vi "Interference 1065.375 Textfile.vi"() -> (3 "Textfile":string[](array[string]))   [LabVIEW 2020, in "EPA 1065.lvlib" / "Interference verificaton 1065-375.lvlib"]
uses:
  Interference verificaton 1065-375.lvlib
  Sprachverwaltung/FGV Aktion Tabelle zerlegen.ctl
  Aktion FGV Interference.ctl
  Seiten/FT-IR/FGV FT-IR Aktionen.ctl
  Aktion Index uebersetzten.ctl
  Seiten/System Einstellungen V2/Aktioen FGV System Konstanten.ctl
  Visualisierungs Elemente/String - Ausgabefeld.ctl
  Seiten/FT-IR/FT-IR.lvlib
  Seiten/System Einstellungen V2/System Einstellungen V2.lvlib
  Sprachverwaltung/Sprachverwaltung.lvlib
panel:
  out "Tabellen-String":string
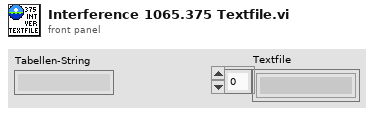
[diagram p1: front panel]
types:
  T1 = typedef "String - Ausgabefeld.ctl" = string
  T2 = typedef "System Einstellungen V2.lvlib/Aktioen FGV System Konstanten.ctl" = enum16{"lesen", "laden", "speichern", "Sprache"}
  T3 = typedef "EPA 1065.lvlib/Interference verificaton 1065-375.lvlib/Aktion Index uebersetzten.ctl" = enum16{"lesen", "schreiben", "auswerten"}
  T4 = typedef "FT-IR.lvlib/FGV FT-IR Aktionen.ctl" = enum16{"lesen", "NOG setzen", "NOS setzen", "Initialisieren", "speichern", "ALLES setzen", "FT-IR Spektrum loggen", "Komm Stoppen", "Spektrum LogKonfig"}
  T5 = typedef "EPA 1065.lvlib/Interference verificaton 1065-375.lvlib/Aktion FGV Interference.ctl" = enum16{"Lesen", "TestKonfig", "TestSetting", "Einheiten", "Ergebnis", "Laden", "Tabelle", "Speichern", "löschen"}
  T6 = typedef "Sprachverwaltung.lvlib/FGV Aktion Tabelle zerlegen.ctl" = enum16{"laden", "vereinzeln", "speichern"}
  T7 = typedef "EPA 1065.lvlib/Interference verificaton 1065-375.lvlib/TestSetting.ctl" = cluster{"Bearbeiter:":string, "Pfad:":path, "Textname:":string, "Analysator":T8}
  T8 = typedef "System Einstellungen V2.lvlib/Analysatoren.ctl" = string
  T9 = typedef "EPA 1065.lvlib/Interference verificaton 1065-375.lvlib/TestKonfig.ctl" = cluster{"Komponente:":u16, "Modus":T10, "CG Aufschaltzeit:":dbl, "Interferent 1:":u16, "Interferent 2:":u16, "Interferent 3:":u16, "Gasflaschen Nr.:":string, "Gasflaschen Nr.: 2":string, "Gasflaschen Nr.: 3":string, "Inter 1 aktiv":bool, "Inter 2 aktiv":bool, "Inter 3 aktiv":bool, "Accuracy":string, "Accuracy 2":string, "Accuracy 3":string, "Konzentration 1:":dbl, "Konzentration 2:":dbl, "Konzentration 3:":dbl}
  T10 = typedef "EPA 1065.lvlib/Interference verificaton 1065-375.lvlib/Modus.ctl" = u16
  T11 = typedef "EPA 1065.lvlib/Interference verificaton 1065-375.lvlib/Komponenten.ctl" = cluster{"Komponente":T1, "Komponente Index":i32, "Komponente 2":T1, "Komponente Index 2":i32, "Komponente 3":T1, "Komponente Index 3":i32, "Interferent 1":T1, "Interferent Index":i32, "Interferent 2":T1, "Interferent 2 Index":i32, "Interferent 3":T1, "Interferent 3 Index":i32, "Interferent 4":T1, "Interferent 4 Index":i32}
  T12 = cluster{"Modell":string, "ProjektNummer":string, "Software Version":string, "Seriennummer":string}
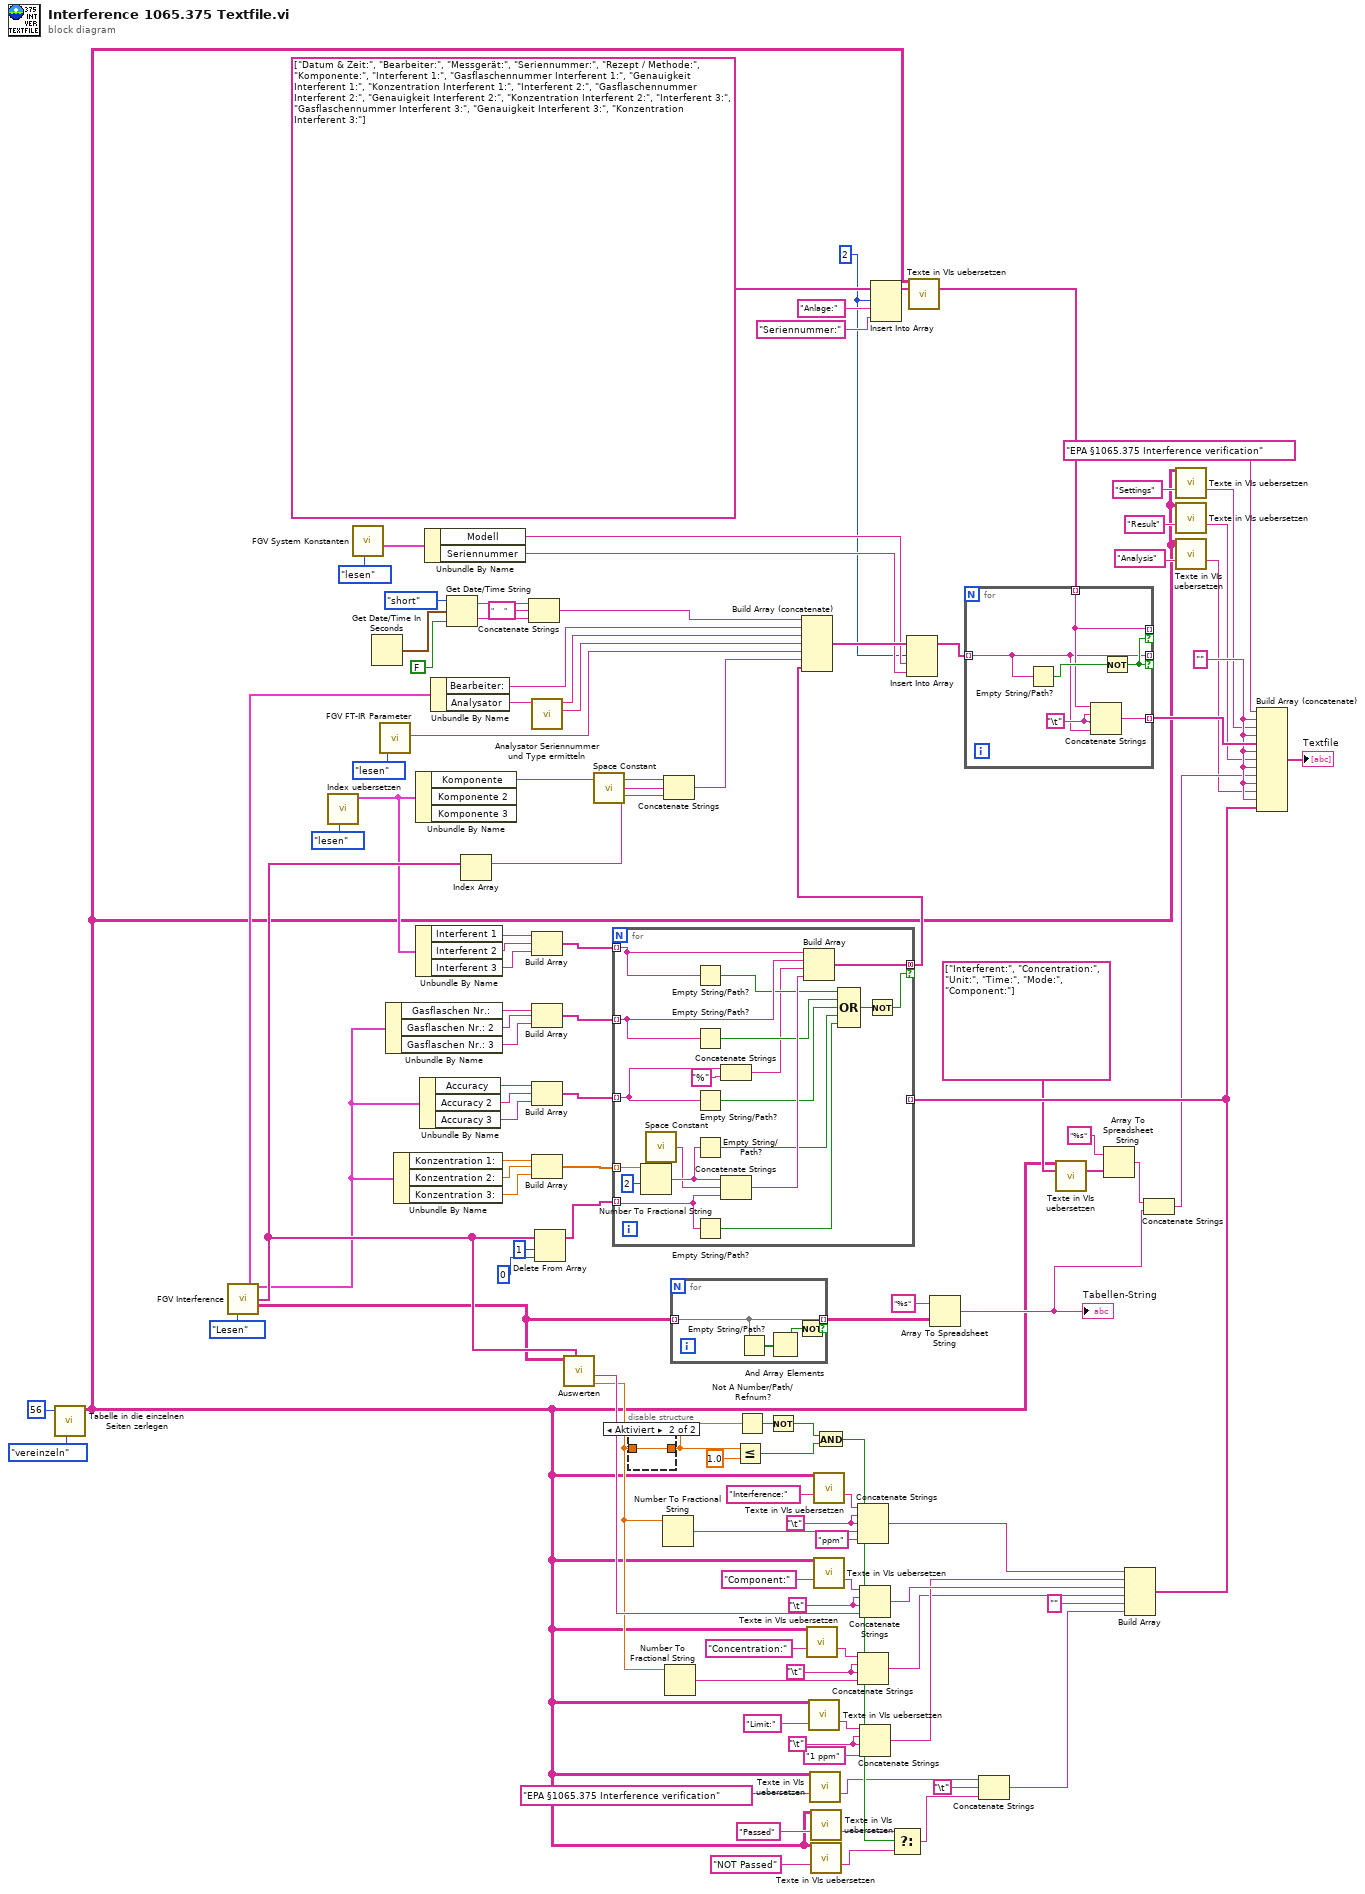
[diagram p0: block diagram]
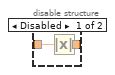
[diagram p2: hidden frame]
diagram:
  w35 = ""
  w52 = "\t"
  w53 = "\t"
  w54 = "\t"
  w55 = "\t"
  w63 = 2 ("Index")
  n1 = call "Tabelle in die einzelnen Seiten zerlegen.vi"("Aktion"=FGV_Aktion_Tabelle_zerlegen."vereinzeln", "Index (Seite)"=56) -> ("Sprachliste"=w4:string[][])  [unwired: 7 in, 2 out]
  n2 = call "FGV Interference.vi"("Aktion FGV Interference"=Aktion_FGV_Interference."Lesen") -> ("TestSetting"=w113:T7, "TestKonfig 2"=w82:T9, "Êinheiten"=w100:string[], "Tabelle"=w32:T1[][])  [unwired: 9 in, 2 out]
  n3 = call "Index uebersetzen.vi"("Aktion"=Aktion_Index_uebersetzten."lesen") -> ("Komponenten"=w95:T11)  [unwired: 9 in, 1 out]
  n4 = call "FGV System Konstanten.vi"("Aktionen"=Aktioen_FGV_System_Konstanten."lesen") -> ("Cluster out"=w72:T12)  [unwired: 6 in, 4 out]
  n5 = Get Date/Time In Seconds() -> (seconds since 1Jan1904=w112:timestamp)
  n6 = call "FGV FT-IR Parameter.vi"("Aktion"=FGV_FT-IR_Aktionen."lesen") -> ("Current Recipe"=w101:string)  [unwired: 11 in, 7 out]
  n7 = Unbundle By Name(w82) -> ("Gasflaschen Nr.:"=w94:string, "Gasflaschen Nr.: 2"=w93:string, "Gasflaschen Nr.: 3"=w92:string)
  n8 = Unbundle By Name(w82) -> ("Konzentration 1:"=w91:dbl, "Konzentration 2:"=w90:dbl, "Konzentration 3:"=w89:dbl)
  n9 = Unbundle By Name(w95) -> ("Komponente"=w75:T1)  [unwired: 2 out]
  n10 = Unbundle By Name(w95) -> ("Interferent 1"=w98:T1, "Interferent 2"=w97:T1, "Interferent 3"=w96:T1)
  n11 = Unbundle By Name(w82) -> ("Accuracy"=w81:string, "Accuracy 2"=w80:string, "Accuracy 3"=w79:string)
  n12 = Unbundle By Name(w72) -> ("Modell"=w65:string, "Seriennummer"=w64:string)
  n13 = Unbundle By Name(w113) -> ("Bearbeiter:"=w103:string, "Analysator"=w3:T8)
  n14 = Get Date/Time String(date format (0)=enum16{"short", "long", "abbreviated"}."short" ("Datumsformat (0)"), seconds (now)=w112, want seconds? (F)=FALSE ("Angabe von Sekunden? (F)")) -> (date string=w111:string, time string=w110:string)
  n15 = Index Array(array=w100) -> (element=w74:string)  [unwired: 1 in]
  n16 = Concatenate Strings(w111, "     " ("String"), w110) -> (w104:string)
  n17 = call "Analysator Seriennummer und Type ermitteln.vi"("Analysator"=w3) -> ("Type"=w2:string, "Name für Protokoll"=w1:string)  [unwired: 8 in, 1 out]
  n18 = Build Array(w98, w97, w96) -> (w88:T1[])
  n19 = Build Array(w94, w93, w92) -> (w87:string[])
  n20 = Build Array(w81, w80, w79) -> (w78:string[])
  n21 = Build Array(w91, w90, w89) -> (w86:dbl[])
  n22 = Delete From Array(array=w100, length=1 ("Länge"), index=0 ("Index")) -> (array with subset deleted=w84:string[])  [unwired: 1 out]
  n23 = call "Auswerten.vi"("Êinheiten"=w100, "Tabelle"=w32) -> ("Konzentration Komponente"=w49:dbl, "Komponente:"=w50:T1)  [unwired: 6 in, 2 out]
  n24 = call <vilib>:"Space Constant.vi"() -> ("String"=w76:string)
  n25 = disable-structure shown="Aktiviert" {
    disable-tunnel: w49 -> [w118 w119]
    disable-tunnel: [w117 w119] -> w45
    frame Disabled {
      n26 = Absolute Value(x=w118) -> (abs(x)=w117:dbl)
    }
    frame Enabled {
    }
  }
  n27 = Number To Fractional String(number=w49) -> (F-format string=w60:string)  [unwired: 3 in]
  n28 = Concatenate Strings(w75, w76, w74) -> (w102:string)
  n29 = Number To Fractional String(number=w49) -> (F-format string=w56:string)  [unwired: 3 in]
  n30 = for {
    tunnel: w32 -> [w123] mode=indexing
    tunnel: [w123] -> w33 mode=indexing if=w120
    n31 = Empty String/Path?(string/path=w123) -> (empty?=w122:bool[])
    n32 = And Array Elements(Boolean array=w122) -> (logical AND=w121:bool)
    n33 = Not(x=w121) -> (.not. x?=w120:bool)
  }
  n34 = Less Or Equal?(x=w45, y=1.0) -> (x <= y?=w43:bool)
  n35 = Not A Number/Path/Refnum?(number/path/refnum=w45) -> (NaN/Path/Refnum?=w44:bool)
  n36 = Not(x=w44) -> (.not. x?=w42:bool)
  n37 = call "Texte in VIs uebersetzen.vi"("Sprachliste"=w4, "String zum Übersetzen"="Concentration:" ("String")) -> ("String zum Übersetzen"=w13:string)  [unwired: 9 in, 4 out]
  n38 = call "Texte in VIs uebersetzen.vi"("Sprachliste"=w4, "String zum Übersetzen"="Limit:" ("String")) -> ("String zum Übersetzen"=w11:string)  [unwired: 9 in, 4 out]
  n39 = call "Texte in VIs uebersetzen.vi"("Sprachliste"=w4, "String zum Übersetzen"="EPA §1065.375 Interference verification") -> ("String zum Übersetzen"=w9:string)  [unwired: 9 in, 4 out]
  n40 = call "Texte in VIs uebersetzen.vi"("Sprachliste"=w4, "String zum Übersetzen"=T1 "Passed" ("String")) -> ("String zum Übersetzen"=w7:string)  [unwired: 9 in, 4 out]
  n41 = call "Texte in VIs uebersetzen.vi"("Sprachliste"=w4, "String zum Übersetzen"=T1 "NOT Passed" ("String")) -> ("String zum Übersetzen"=w5:string)  [unwired: 9 in, 4 out]
  n42 = call "Texte in VIs uebersetzen.vi"("Sprachliste"=w4, "String zum Übersetzen"="Interference:" ("String")) -> ("String zum Übersetzen"=w17:string)  [unwired: 9 in, 4 out]
  n43 = call "Texte in VIs uebersetzen.vi"("Sprachliste"=w4, "String zum Übersetzen"="Component:" ("String")) -> ("String zum Übersetzen"=w15:string)  [unwired: 9 in, 4 out]
  n44 = And(x=w42, y=w43) -> (x .and. y?=w61:bool)
  n45 = Concatenate Strings(w17, w55, w55, w60, "ppm" ("String")) -> (w58:string)
  n46 = Concatenate Strings(w13, w53, w53, w56) -> (w39:string)
  n47 = Concatenate Strings(w15, w54, w54, w50) -> (w57:string)
  n48 = Concatenate Strings(w11, w52, w52, "1 ppm" ("String")) -> (w40:string)
  n49 = Insert Into Array(array=string[] ["Datum & Zeit:", "Bearbeiter:", "Messgerät:", "Seriennummer:", "Rezept / Methode:", "Komponente:", "Interferent 1:", "Gasflaschennummer Interferent 1:", "Genauigkeit Interferent 1:", "Konzentration Interferent 1:", "Interferent 2:", "Gasflaschennummer Interferent 2:", "Genauigkeit Interferent 2:", "Konzentration Interferent 2:", "Interferent 3:", "Gasflaschennummer Interferent 3:", "Genauigkeit Interferent 3:", "Konzentration Interferent 3:"], index=w63, new element #1="Anlage:" ("Neues Element/Teil-Array"), new element #2="Seriennummer:" ("Neues Element/Teil-Array")) -> (w68:string[])
  n50 = Select(t=w7, s=w61, f=w5) -> (s? t:f=w19:string)
  n51 = call "Texte in VIs uebersetzen.vi"("Sprachliste"=w4, "String-Array zum Übersetzen"=w68) -> ("String-Array zum Übersetzen"=w77:string[])  [unwired: 9 in, 4 out]
  n52 = Array To Spreadsheet String(array=w33, 3:"%s" ("Format-String")) -> (spreadsheet string=w29:string)  [unwired: 1 in]
  "Tabellen-String" <- w29
  n53 = Concatenate Strings(w9, "\t", w19) -> (w37:string)
  n54 = call "Texte in VIs uebersetzen.vi"("Sprachliste"=w4, "String-Array zum Übersetzen"=string[] ["Interferent:", "Concentration:", "Unit:", "Time:", "Mode:", "Component:"]) -> ("String-Array zum Übersetzen"=w20:string[])  [unwired: 9 in, 4 out]
  n55 = Array To Spreadsheet String(array=w20, 3:"%s" ("Format-String")) -> (spreadsheet string=w30:string)  [unwired: 1 in]
  n56 = Build Array(w58, w40, w57, w39, "" ("Element"), w37) -> (w48:string[])
  n57 = for {
    tunnel: w88 -> [w139] mode=indexing
    tunnel: w87 -> [w138] mode=indexing
    tunnel: w86 -> [w142] mode=indexing
    tunnel: w84 -> [w141] mode=indexing
    tunnel: [w136] -> w83 mode=concatenating if=w124
    tunnel: w78 -> [w125] mode=indexing
    tunnel: w48 -> [_] mode=indexing
    n58 = Number To Fractional String(number=w142, precision (6)=i16 2 ("Genauigkeit (6)")) -> (F-format string=w140:string)  [unwired: 2 in]
    n59 = call <vilib>:"Space Constant.vi"() -> ("String"=w130:string)
    n60 = Empty String/Path?(string/path=w139) -> (empty?=w135:bool)
    n61 = Empty String/Path?(string/path=w138) -> (empty?=w134:bool)
    n62 = Empty String/Path?(string/path=w125) -> (empty?=w126:bool)
    n63 = Empty String/Path?(string/path=w140) -> (empty?=w131:bool)
    n64 = Empty String/Path?(string/path=w141) -> (empty?=w133:bool)
    n65 = Concatenate Strings(w125, "%" ("String")) -> (w128:string)
    n66 = Concatenate Strings(w140, w130, w141) -> (w137:string)
    n67 = Build Array(w139, w138, w128, w137) -> (w136:T1[])
    n68 = Compound Arithmetic op=OR ("Mehrfacharithmetik")(w135, w134, w126, w131, w133) -> (w132:bool)
    n69 = Not(x=w132) -> (.not. x?=w124:bool)
  }
  n70 = Build Array (concatenate)(w104, w103, w1, w2, w101, w102, w83) -> (w67:T1[])
  n71 = Insert Into Array(array=w67, index=w63, new element #1=w65, new element #2=w64) -> (w66:T1[])
  n72 = for {
    tunnel: w66 -> [w144] mode=indexing
    tunnel: [w144] -> _ mode=indexing if=w147
    tunnel: [w145] -> _ mode=indexing if=w147
    tunnel: w77 -> [w145] mode=indexing
    tunnel: [w143] -> w36 mode=indexing
    w146 = "\t"
    n73 = Empty String/Path?(string/path=w144) -> (empty?=w148:bool)
    n74 = Concatenate Strings(w145, w146, w146, w144) -> (w143:string)
    n75 = Not(x=w148) -> (.not. x?=w147:bool)
  }
  n76 = Concatenate Strings(w30, w29) -> (w28:string)
  n77 = call "Texte in VIs uebersetzen.vi"("Sprachliste"=w4, "String zum Übersetzen"="Settings" ("Element")) -> ("String zum Übersetzen"=w26:string)  [unwired: 9 in, 4 out]
  n78 = call "Texte in VIs uebersetzen.vi"("Sprachliste"=w4, "String zum Übersetzen"="Result" ("Element")) -> ("String zum Übersetzen"=w24:string)  [unwired: 9 in, 4 out]
  n79 = call "Texte in VIs uebersetzen.vi"("Sprachliste"=w4, "String zum Übersetzen"="Analysis" ("Element")) -> ("String zum Übersetzen"=w22:string)  [unwired: 9 in, 4 out]
  n80 = Build Array (concatenate)("EPA §1065.375 Interference verification", w35, w26, w35, w36, w35, w24, w35, w28, w35, w22, w35, w48) -> (→"Textfile":string[])
